vi "Write Group Metadata.vi"(0 "reference in":refnum<class "TDMS_DataHandler.lvclass">, 5 "error in (no error)":errorcluster) -> (14 "reference out":refnum<class "TDMS_DataHandler.lvclass">, 16 "group name out":string, 17 "channel name out":string, 19 "error out":errorcluster)   [LabVIEW 2019, in "TDMS_DataHandler.lvclass"]
doc: "Write the metadata of the given channel of the tdms file"
uses:
  TDMS_DataHandler.lvclass
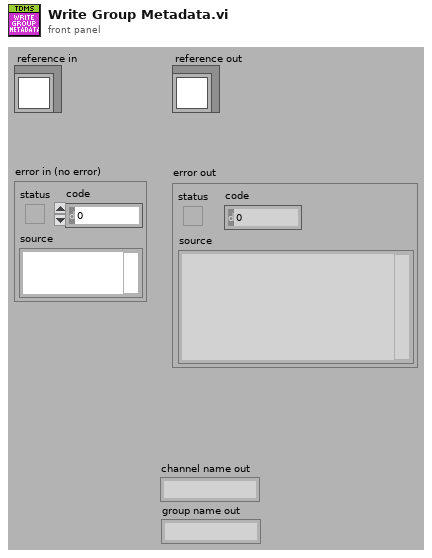
[diagram p1: front panel]
types:
  T1 = typedef "TDMS_DataHandler.lvclass/ObjectAttributes.ctl" = cluster{"Directory":path, "FilePath":path, "FileRef":refnum<k34>, "ExperimentName":string, "GroupName":string, "ChannelNames":string[], "Datum":waveform(dbl)[], "Group_Metadata":cluster{"property names":string[], "property values":variant[]}, "Channel_Metadata":cluster{"property names":string[], "property values":variant[]}}
  T2 = cluster{"property names":string[], "property values":variant[]}
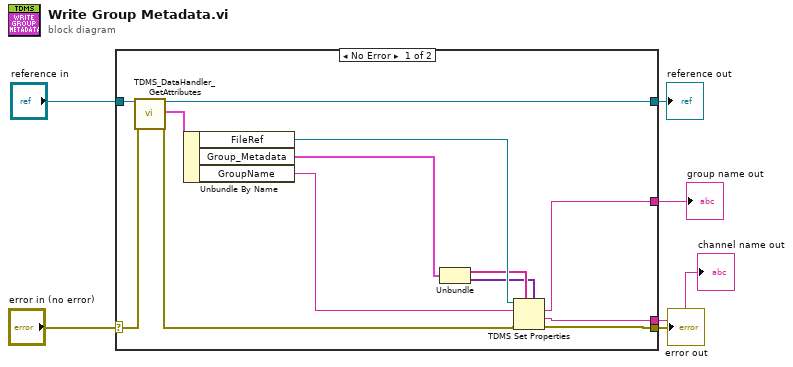
[diagram p0: block diagram]
diagram:
  n1 = case shown="No Error" "error in (no error)" {
    selector: "error in (no error)" -> [w19 w21]
    tunnel: [w8 w21] -> w5
    tunnel: [w18 w20] -> w3
    tunnel: "reference in" -> [w16 w20]
    tunnel: [w11 _] -> w2
    tunnel: [w10 _] -> w1
    frame No Error {
      n2 = call "TDMS_DataHandler_GetAttributes.vi"("reference in"=w16, "error in (no error)"=w19) -> ("reference out"=w18:refnum<class "TDMS_DataHandler.lvclass">, "attributes"=w17:T1, "error out"=w9:errorcluster)  [unwired: 14 in, 1 out]
      n3 = Unbundle By Name(w17) -> ("FileRef"=w15:refnum<k34>, "Group_Metadata"=w14:T2, "GroupName"=w7:string)
      n4 = Unbundle(w14) -> ("property names"=w13:string[], "property values"=w12:variant[])
      n5 = TDMS Set Properties(5:w12, 7:w13, 8:w9, 10:w7, 11:w15) -> (0:w8:errorcluster, 1:w11:string, 2:w10:string)  [unwired: 1 in, 1 out]
    }
    frame Error {
    }
  }
  "error out" <- w5
  "reference out" <- w3
  "channel name out" <- w2
  "group name out" <- w1
